vi "Dialog.vi"(8 "error in (no error)":errorcluster, 10 "button name (\"OK\")":string="OK", 11 "message":string) -> (0 "error out":errorcluster)   [LabVIEW 2014]
panel:
  # "LICENSED MATERIALS – PROPERTY OF IBM\nCopyright IBM Corp. 2016,\nALL RIGHTS RESERVED"
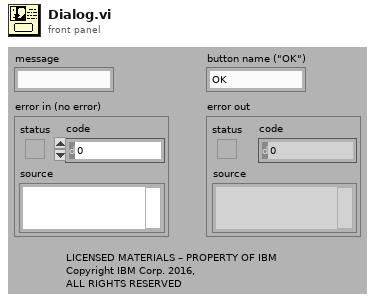
[diagram p1: front panel]
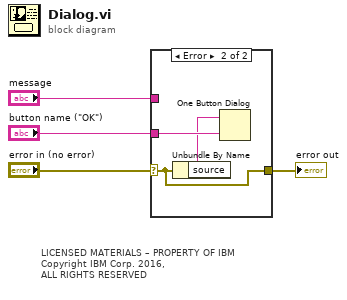
[diagram p0: block diagram]
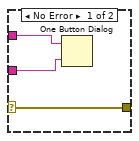
[diagram p2: hidden frame]
diagram:
  # "LICENSED MATERIALS – PROPERTY OF IBM\nCopyright IBM Corp. 2016,\nALL RIGHTS RESERVED"
  n1 = case shown="Error" "error in (no error)" {
    selector: "error in (no error)" -> [w5 w8]
    tunnel: "message" -> [w7 _]
    tunnel: "button name (\"OK\")" -> [w6 w10]
    tunnel: [w5 w8] -> w2
    frame No Error {
      n2 = One Button Dialog(message=w7, button name ("OK")=w6) -> ()  [unwired: 1 out]
    }
    frame Error {
      n3 = Unbundle By Name(w8) -> ("source"=w9:string)
      n4 = One Button Dialog(message=w9, button name ("OK")=w10) -> ()  [unwired: 1 out]
    }
  }
  "error out" <- w2
